vi "InsertSubpanel.vi"(8 "error in (no error)":errorcluster, 9 "Subpanel":i32, 10 "Panel":i32, 11 "Maui Manager in":refnum<class "Maui Manager.lvclass">) -> (0 "error out":errorcluster, 3 "Maui Manager out":refnum<class "Maui Manager.lvclass">)   [LabVIEW 2019, in "Maui Manager.lvclass"]
uses:
  Maui Manager.lvclass
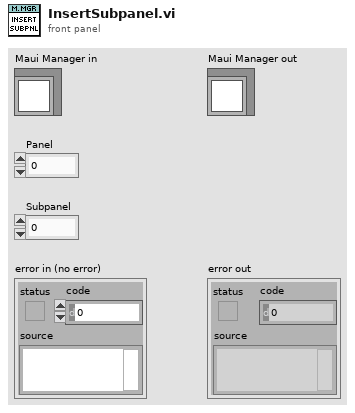
[diagram p1: front panel]
types:
  T1 = cluster{"Control":refnum<vi>, "Subpanel":refnum<vi>, "Active":i32, "Ctrl Class":string}[]
  T2 = enum32{"Invalid", "Standard", "Closed", "Hidden", "Minimized", "Maximized"}
  T3 = cluster{"Control":refnum<vi>, "Subpanel":refnum<vi>, "Active":i32, "Ctrl Class":string}
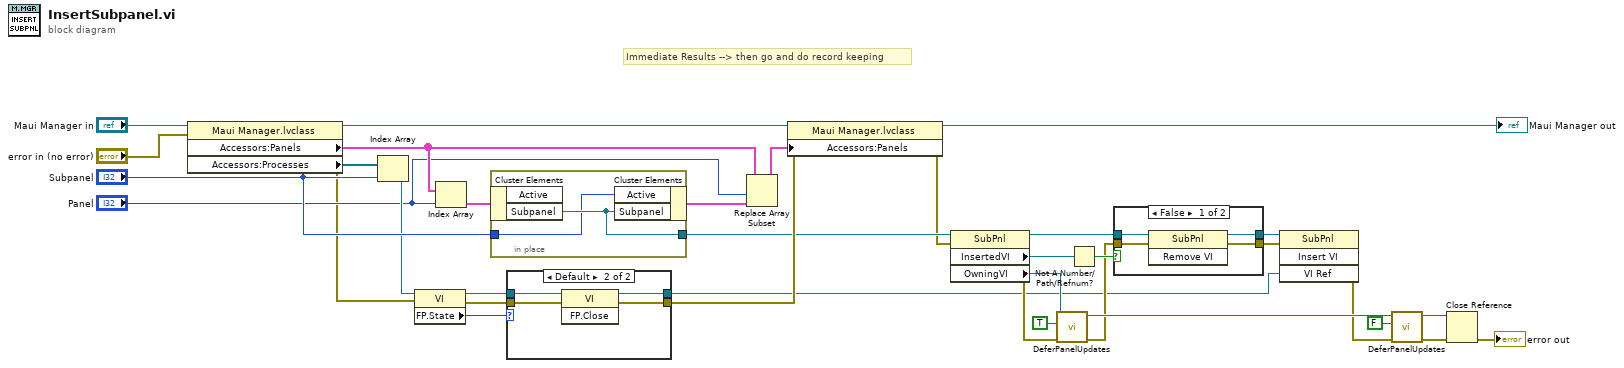
[diagram p0: block diagram]
diagram:
  # "Immediate Results --> then go and do record keeping"
  n1 = property class="Maui Manager.lvclass"(reference="Maui Manager in", error in="error in (no error)") -> (reference out=w34:refnum<class "Maui Manager.lvclass">, error out=w20:errorcluster, "Accessors:Panels"=w23:T1, "Accessors:Processes"=w31:refnum<vi>[])
  n2 = Index Array(array=w31, index="Subpanel") -> (element=w28:refnum<vi>)
  n3 = property class="VI"(reference=w28, error in=w20) -> (reference out=w27:refnum<vi>, error out=w25:errorcluster, "FP.State"=w26:T2)
  n4 = Index Array(array=w23, index="Panel") -> (element=w30:T3)
  n5 = in-place {
    in-place-border: [w37] -> w18
    in-place-border: "Subpanel" -> [w36]
    n6 = in-place-cluster #1(w30) -> ("Subpanel"=w37:refnum<vi>)  [unwired: 1 out]
    n7 = in-place-cluster #1("Active"=w36, "Subpanel"=w37) -> (w22:T3)
  }
  n8 = case shown="Default" w26 {
    tunnel: w27 -> [w39 w43]
    tunnel: [w39 w42] -> w2
    tunnel: [w38 w40] -> w19
    tunnel: w25 -> [w38 w41]
    frame "Closed" {
    }
    frame Default {
      n9 = invoke class="VI" method="FP.Close"(reference=w43, error in=w41) -> (reference out=w42:refnum<vi>, error out=w40:errorcluster)  [unwired: 1 in, 1 out]
    }
  }
  n10 = Replace Array Subset(array=w23, new element=w22, index="Panel") -> (w24:T1)
  n11 = property class="Maui Manager.lvclass"(reference=w34, error in=w19, "Accessors:Panels"=w24) -> (reference out=→"Maui Manager out":refnum<class "Maui Manager.lvclass">, error out=w14:errorcluster)
  n12 = property class="SubPnl"(reference=w18, error in=w14) -> (reference out=w15:refnum<vi>, error out=w8:errorcluster, "InsertedVI"=w17:refnum<vi>, "OwningVI"=w5:refnum<vi>)
  n13 = call "DeferPanelUpdates.vi"("error in (no error)"=w8, "Defer Panel Updates"=TRUE, "VI Refnum In"=w5) -> ("error out"=w7:errorcluster, "VI Refnum Out"=w10:refnum<vi>)  [unwired: 7 in]
  n14 = Not A Number/Path/Refnum?(number/path/refnum=w17) -> (NaN/Path/Refnum?=w16:bool)
  n15 = case shown="False" w16 {
    tunnel: w15 -> [w47 w48]
    tunnel: [w46 w48] -> w12
    tunnel: w7 -> [w45 w49]
    tunnel: [w44 w49] -> w11
    frame False {
      n16 = invoke class="SubPnl" method="Remove VI"(reference=w47, error in=w45) -> (reference out=w46:refnum<vi>, error out=w44:errorcluster)  [unwired: 1 in, 1 out]
    }
    frame True {
    }
  }
  n17 = invoke class="SubPnl" method="Insert VI"(reference=w12, error in=w11, "VI Ref"=w2) -> (error out=w6:errorcluster)  [unwired: 1 in, 3 out]
  n18 = call "DeferPanelUpdates.vi"("error in (no error)"=w6, "Defer Panel Updates"=FALSE, "VI Refnum In"=w10) -> ("error out"=w3:errorcluster, "VI Refnum Out"=w4:refnum<vi>)  [unwired: 7 in]
  n19 = Close Reference(reference=w4, error in (no error)=w3) -> (error out=→"error out":errorcluster)
